vi "ReadWrite.ProcessData.Buffer.vi"(8 "error in (no error)":errorcluster, 9 "Offset":i32, 10 "Values":dbl[](array[numeric]), 11 "ReadWrite in":refnum<class "ReadWrite.lvclass">) -> (0 "error out":errorcluster, 3 "ReadWrite out":refnum<class "ReadWrite.lvclass">)   [LabVIEW 2027, in "Data Access Engine.lvlib" / "ReadWrite.lvclass"]
uses:
  ReadWrite.lvclass
  ReadWrite.lvclass/ReadWrite.ctl
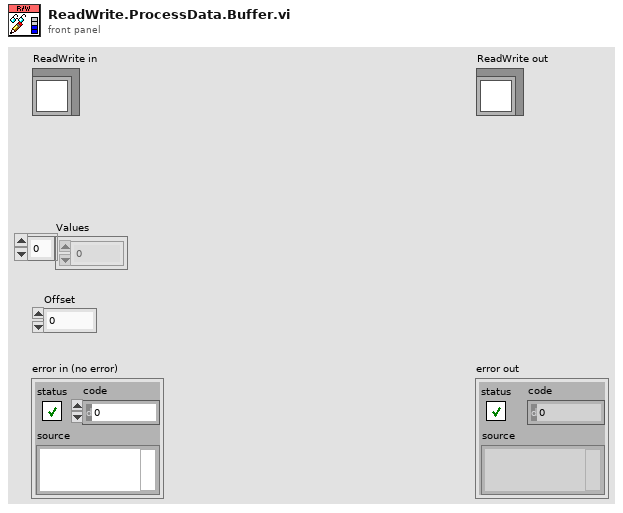
[diagram p1: front panel]
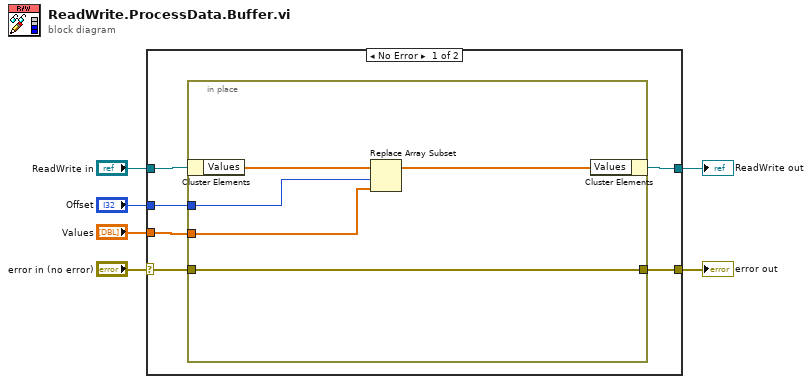
[diagram p0: block diagram]
diagram:
  n1 = case shown="No Error" "error in (no error)" {
    selector: "error in (no error)" -> [w12 w19]
    tunnel: [w7 w19] -> w5
    tunnel: [w10 w18] -> w3
    tunnel: "ReadWrite in" -> [w11 w18]
    tunnel: "Values" -> [w9 _]
    tunnel: "Offset" -> [w8 _]
    frame No Error {
      n2 = in-place {
        in-place-border: w12 -> [w13]
        in-place-border: w9 -> [w17]
        in-place-border: w8 -> [w16]
        in-place-border: [w13] -> w7
        n3 = in-place-cluster #1(w11) -> ("Values"=w15:dbl[])
        n4 = Replace Array Subset(array=w15, new element=w17, index=w16) -> (w14:dbl[])
        n5 = in-place-cluster #1("Values"=w14) -> (w10:refnum<class "ReadWrite.lvclass">)
      }
    }
    frame Error {
    }
  }
  "error out" <- w5
  "ReadWrite out" <- w3
